vi "finishKickoffEnemyPlayVSS.vi"(8 "error in (no error)":errorcluster, 10 "Game in":refnum<class "Game.lvclass">, 11 "KickoffEnemyPlayVSS in":refnum<class "KickoffEnemyPlayVSS.lvclass">) -> (0 "error out":errorcluster, 2 "result":bool, 3 "KickoffEnemyPlayVSS out":refnum<class "KickoffEnemyPlayVSS.lvclass">)   [LabVIEW 2023, in "KickoffEnemyPlayVSS.lvclass"]
uses:
  KickoffEnemyPlayVSS.lvclass
  Game_class/Game.lvclass
  Command.ctl
  Game_class/Game.lvclass/Game.ctl
  Events_class/Events.lvclass/Events.ctl
  Game_class/Read Referee.vi
  Game_class/Read EventsRef.vi
  Events_class/Read touch.vi
  Referee_class/Referee.lvclass
  Events_class/Events.lvclass
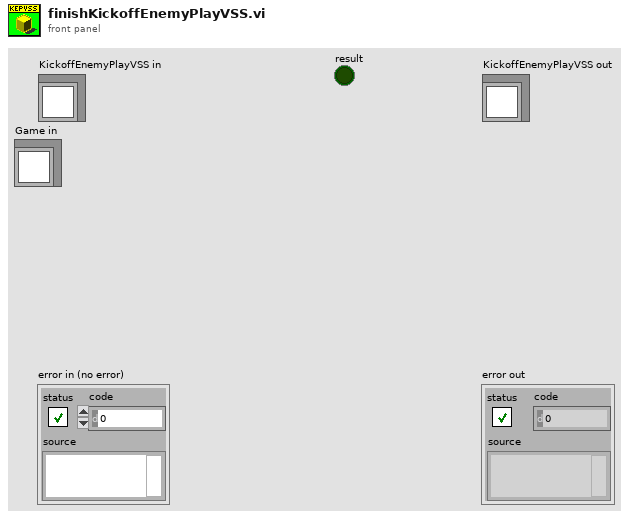
[diagram p1: front panel]
types:
  T1 = typedef "Command.ctl" = enum16{"AUTO", "GAME_ON", "STOP", "HALT", "KICKOFF_ALLY", "KICKOFF_ENEMY", "FREE_BALL", "GOAL_KICK_ENEMY", "GOAL_KICK_ALLY", "PENALTY_KICK_ENEMY", "PENALTY_KICK_ALLY", "FREE_KICK"}
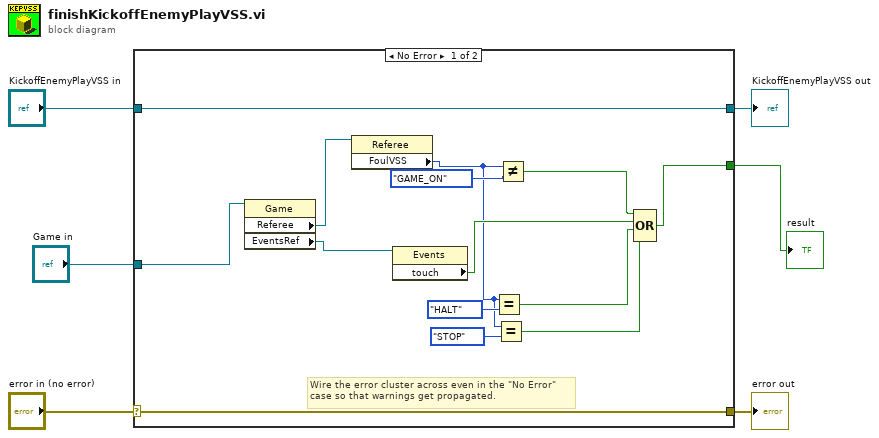
[diagram p0: block diagram]
diagram:
  n1 = case shown="No Error" "error in (no error)" {
    selector: "error in (no error)" -> [w19 w22]
    tunnel: [w19 w22] -> w5
    tunnel: [w20 w21] -> w3
    tunnel: "KickoffEnemyPlayVSS in" -> [w20 w21]
    tunnel: "Game in" -> [w18 _]
    tunnel: [w14 _] -> w1
    frame No Error {
      # "Wire the error cluster across even in the \"No Error\"\ncase so that warnings get propagated."
      n2 = property class="Game"(reference=w18) -> ("Referee"=w17:refnum<class "Referee.lvclass">, "EventsRef"=w15:refnum<class "Events.lvclass">)  [unwired: 1 in, 2 out]
      n3 = property class="Referee"(reference=w17) -> ("FoulVSS"=w9:T1)  [unwired: 1 in, 2 out]
      n4 = property class="Events"(reference=w15) -> ("touch"=w16:bool)  [unwired: 1 in, 2 out]
      n5 = Equal?(x=w9, y=Command."HALT") -> (x = y?=w12:bool)
      n6 = Equal?(x=w9, y=Command."STOP") -> (x = y?=w7:bool)
      n7 = Not Equal?(x=w9, y=Command."GAME_ON") -> (x != y?=w10:bool)
      n8 = Compound Arithmetic op=OR(w10, w16, w12, w7) -> (w14:bool)
    }
    frame Error {
    }
  }
  "error out" <- w5
  "KickoffEnemyPlayVSS out" <- w3
  "result" <- w1
